vi "DSF.Shared.Configuration.Transfer.Create.vi"(8 "error in (no error)":errorcluster, 11 "Transfer Configuration cluster":T1) -> (0 "error out":errorcluster, 3 "Transfer Configuration out":refnum<class "DSF.Shared.Configuration.Transfer.lvclass">)   [LabVIEW 2017, in "DSF.Engine.lvlib" / "DSF.Shared.Configuration.Transfer.lvclass"]
uses:
  DSF.Shared.Configuration.Transfer.lvclass
  DSF Configuration API/1.0.0/Public/Controls/DSF Engine Transfer Configuration.ctl
  DSF Configuration API/1.0.0/Public/Controls/DSF Byte Order.ctl
  DSF Configuration API/1.0.0/Public/Controls/DSF Engine Channel Configuration.ctl
  DSF Configuration API/1.0.0/Public/Controls/DSF Data Type.ctl
  DSF Configuration API/1.0.0/Public/Controls/DSF Settings Info.ctl
  DSF.Shared.Configuration.Transfer.lvclass/DSF.Shared.Configuration.Transfer.ctl
  Typedefs/DSF Runtime Channel Block.ctl
  DSF.Engine.lvlib
  DSF Configuration API/1.0.0/DSF Configuration API.lvlib
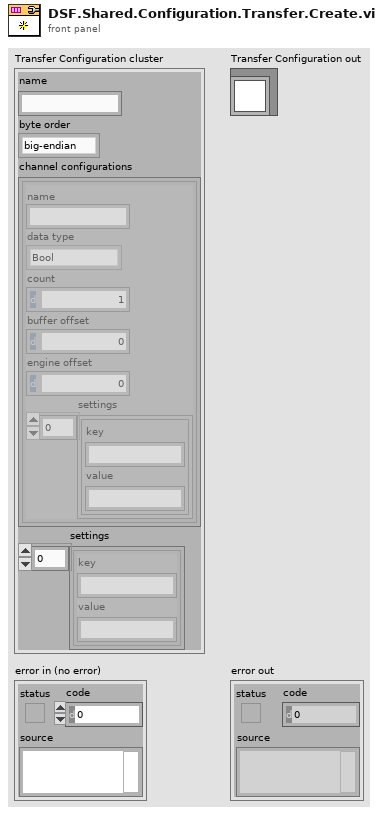
[diagram p1: front panel]
types:
  T1 = typedef "DSF Configuration API.lvlib/DSF Engine Transfer Configuration.ctl" = cluster{"name":string, "byte order":T2, "channel configurations":T3[], "settings":T5}
  T2 = typedef "DSF Configuration API.lvlib/DSF Byte Order.ctl" = enum8{"big-endian", "little-endian"}
  T3 = typedef "DSF Configuration API.lvlib/DSF Engine Channel Configuration.ctl" = cluster{"name":string, "data type":T4, "count":u64, "buffer offset":u64, "engine offset":u64, "settings":T5}
  T4 = typedef "DSF Configuration API.lvlib/DSF Data Type.ctl" = enum8{"Bool", "SGL", "DBL", "I8", "I16", "I32", "I64", "U8", "U16", "U32", "U64"}
  T5 = typedef "DSF Configuration API.lvlib/DSF Settings Info.ctl" = cluster{"key":string, "value":string}[]
  T6 = typedef "DSF.Engine.lvlib/DSF Runtime Channel Block.ctl" = cluster{"data type":T4, "count":u64, "buffer offset":u64}
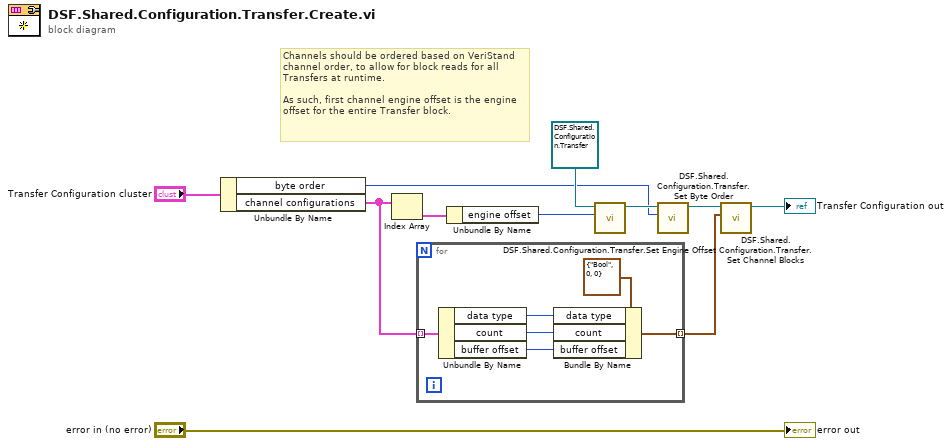
[diagram p0: block diagram]
diagram:
  # "Channels should be ordered based on VeriStand channel order, to allow for block reads for all Transfers at runtime.\n\nAs such, first channel engine offset is the engine offset for the entire Transfer block."
  n1 = Unbundle By Name("Transfer Configuration cluster") -> ("byte order"=w2:T2, "channel configurations"=w8:T3[])
  n2 = Index Array(array=w8) -> (element=w9:T3)  [unwired: 1 in]
  n3 = for {
    tunnel: w8 -> [w16] mode=indexing
    tunnel: [w12] -> w5 mode=indexing
    n4 = Unbundle By Name(w16) -> ("data type"=w15:T4, "count"=w14:u64, "buffer offset"=w13:u64)
    n5 = Bundle By Name(cluster=T6 {"data type"=enum."Bool", "count"=0, "buffer offset"=0} ("Channel Block"), "data type"=w15, "count"=w14, "buffer offset"=w13) -> (w12:T6)
  }
  n6 = Unbundle By Name(w9) -> ("engine offset"=w10:u64)
  n7 = call "DSF.Shared.Configuration.Transfer.Set Engine Offset.vi"("engine offset"=w10, "Transfer Configuration in"=refnum<class "DSF.Shared.Configuration.Transfer.lvclass"> refnum) -> ("Transfer Configuration out"=w4:refnum<class "DSF.Shared.Configuration.Transfer.lvclass">)  [unwired: 9 in]
  n8 = call "DSF.Shared.Configuration.Transfer.Set Byte Order.vi"("byte order"=w2, "Transfer Configuration in"=w4) -> ("Transfer Configuration out"=w7:refnum<class "DSF.Shared.Configuration.Transfer.lvclass">)  [unwired: 9 in]
  n9 = call "DSF.Shared.Configuration.Transfer.Set Channel Blocks.vi"("channel blocks"=w5, "Transfer Configuration in"=w7) -> ("Transfer Configuration out"=→"Transfer Configuration out":refnum<class "DSF.Shared.Configuration.Transfer.lvclass">)  [unwired: 9 in]
  "error out" <- "error in (no error)"
